vi "LoadSysConfig.vi"(8 "Error In":errorcluster, 11 "Enum":enum16{"LastUse", "Default"}(ring)) -> (0 "Error Out":errorcluster, 3 "SysConfigCluster":T1)   [LabVIEW 2020]
uses:
  <userlib>/_OpenG.lib/file/file.llb/openg_file.lvlib
panel:
  out "loading path":path
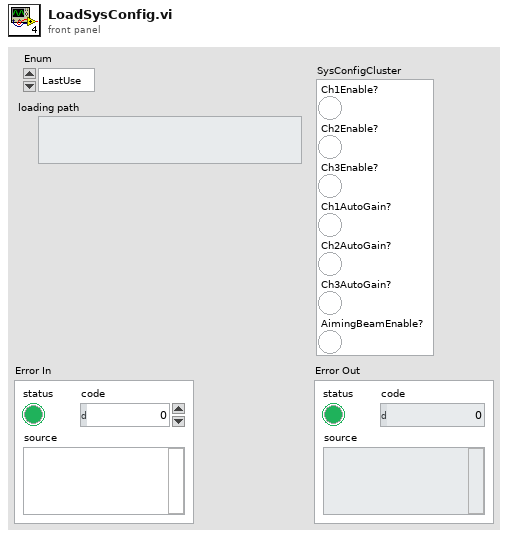
[diagram p1: front panel]
types:
  T1 = cluster{"Ch1Enable?":bool, "Ch2Enable?":bool, "Ch3Enable?":bool, "Ch1AutoGain?":bool, "Ch2AutoGain?":bool, "Ch3AutoGain?":bool, "AimingBeamEnable?":bool}
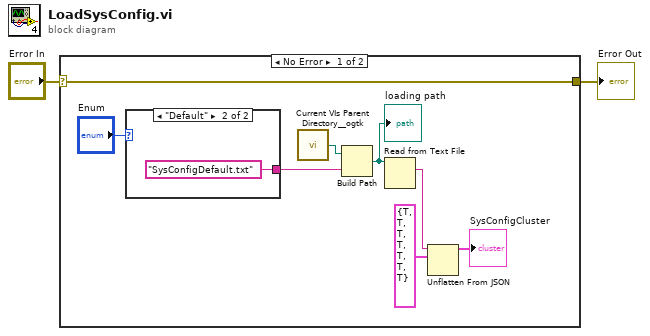
[diagram p0: block diagram]
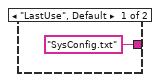
[diagram p2: hidden frame]
diagram:
  n1 = case shown="No Error" "Error In" {
    selector: "Error In" -> [w3 w13]
    tunnel: [w3 w13] -> w1
    frame No Error {
      n2 = case shown="\"Default\"" "Enum" {
        tunnel: ["SysConfig.txt" ("name or relative path") "SysConfigDefault.txt" ("name or relative path")] -> w5
        frame "LastUse", Default {
        }
        frame "Default" {
        }
      }
      n3 = call <userlib>:"Current VIs Parent Directory__ogtk.vi"() -> ("Parent Directory (+ Relative)"=w6:path)  [unwired: 5 in]
      n4 = Build Path(base path=w6, name or relative path=w5) -> (appended path=w7:path)
      "loading path" <- w7
      n5 = Read from Text File(file (use dialog)=w7) -> (text=w8:string)  [unwired: 3 in, 3 out]
      n6 = Unflatten From JSON(JSON string=w8, type and defaults=T1 {"Ch1Enable?"=TRUE, "Ch2Enable?"=TRUE, "Ch3Enable?"=TRUE, "Ch1AutoGain?"=TRUE, "Ch2AutoGain?"=TRUE, "Ch3AutoGain?"=TRUE, "AimingBeamEnable?"=TRUE} ("SysConfigCluster")) -> (value=→"SysConfigCluster":T1)  [unwired: 5 in, 1 out]
    }
    frame Error {
    }
  }
  "Error Out" <- w1
